vi "Array Variant to Key List.vi"(5 "section":string, 7 "Prefix":string, 8 "Error In":errorcluster, 10 "Label.Text":string, 11 "Variant":variant) -> (0 "Error Out":errorcluster, 2 "Key list":T1)   [LabVIEW 2015]
uses:
  <vilib>/Utility/Data Type/NI_Data Type.lvlib
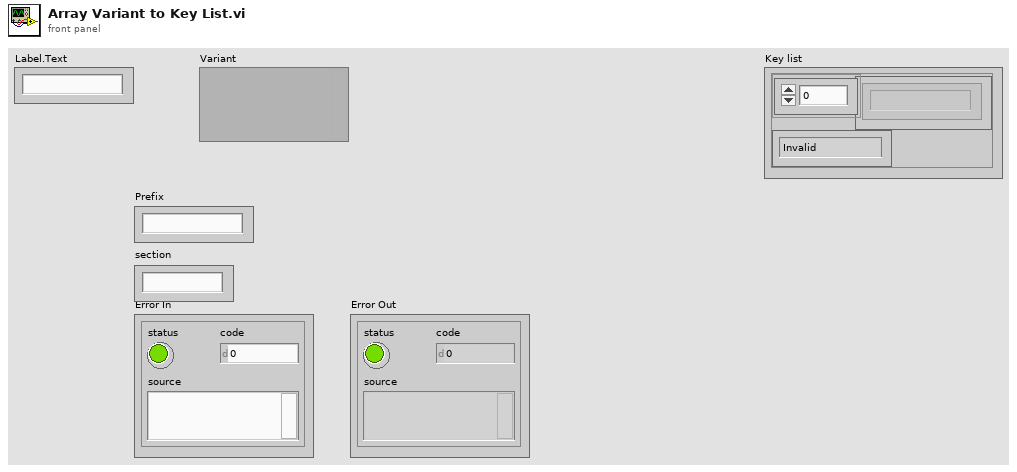
[diagram p1: front panel]
types:
  T1 = cluster{"Array":string[], "Enum":enum16{"Invalid", "Boolean", "Double", "I32", "Path", "String", "U32", "Array", "Cluster"}}
  T2 = typedef "NI_Data Type.lvlib/Data Type.ctl" = enum8{"Invalid Type", "Void", "I8", "I16", "I32", "I64", "U8", "U16", "U32", "U64", "Single Float", "Double Float", "Extended Float", "Single Complex", "Double Complex", "Extended Complex", "Enum U8", "Enum U16", "Enum U32", "Enum U64", "Single Float With Unit", "Double Float With Unit", "Extended Float With Unit", "Single Complex with Unit", "Double Complex with Unit", "Extended Complex with Unit", "Boolean", "String", "Path", "Picture", "Tag", "Array", "Cluster", "Variant", "LV Variant", "Waveform", "Timestamp", "Digital Waveform", "Digital Data", "ExpressData", "Refnum", "External Data", "VI", "Poly VI", "LabVIEW Class Instance", "Fixed Point"}
  T3 = enum16{"Invalid", "Boolean", "Double", "I32", "Path", "String", "U32", "Array", "Cluster"}
  T4 = cluster{string[], enum16{"Invalid", "Boolean", "Double", "I32", "Path", "String", "U32", "Array", "Cluster"}}
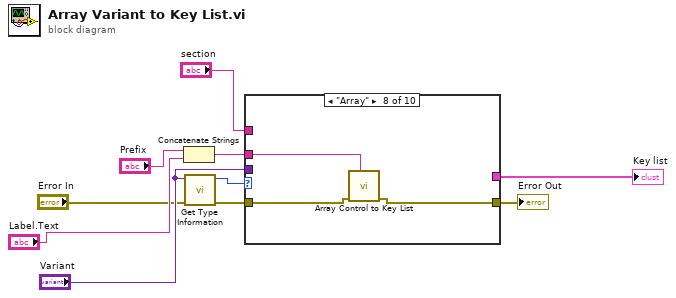
[diagram p0: block diagram]
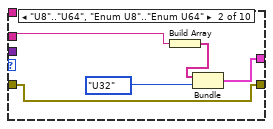
[diagram p3: hidden frame]
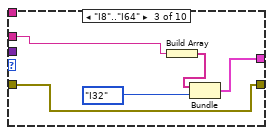
[diagram p4: hidden frame]
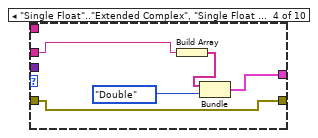
[diagram p5: hidden frame]
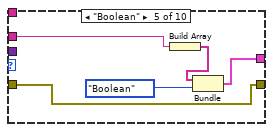
[diagram p6: hidden frame]
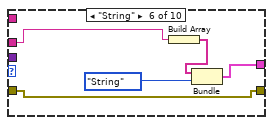
[diagram p7: hidden frame]
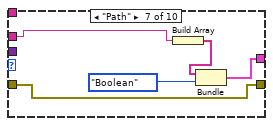
[diagram p8: hidden frame]
diagram:
  n1 = Concatenate Strings("Prefix", "Label.Text") -> (w7:string)
  n2 = call <vilib>:"Get Type Information.vi"("error in (no error)"="Error In", "Variant"="Variant") -> ("error out"=w6:errorcluster, "Type"=w10:T2)  [unwired: 5 in, 3 out]
  n3 = case shown="\"Array\"" w10 {
    tunnel: "section" -> [_ _ _ _ _ _ _ _ _ _]
    tunnel: w7 -> [_ w14 w17 w22 w31 w33 w37 w43 _ _]
    tunnel: w6 -> [w11 w12 w19 w24 w28 w34 w39 w44 _ _]
    tunnel: [w11 w12 w19 w24 w28 w34 w39 w42 _ _] -> w5
    tunnel: "Variant" -> [_ _ _ _ _ _ _ _ _ _]
    tunnel: [_ w13 w18 w23 w27 w32 w38 _ _ _] -> w4
    frame "Invalid Type", Default {
    }
    frame "U8".."U64", "Enum U8".."Enum U64" {
      n4 = Build Array(w14) -> (w16:string[])
      n5 = Bundle(w16, T3."U32") -> (w13:T4)  [unwired: 1 in]
    }
    frame "I8".."I64" {
      n6 = Build Array(w17) -> (w21:string[])
      n7 = Bundle(w21, T3."I32") -> (w18:T4)  [unwired: 1 in]
    }
    frame "Single Float".."Extended Complex", "Single Float With Unit".."Extended Complex with Unit" {
      n8 = Build Array(w22) -> (w26:string[])
      n9 = Bundle(w26, T3."Double") -> (w23:T4)  [unwired: 1 in]
    }
    frame "Boolean" {
      n10 = Build Array(w31) -> (w30:string[])
      n11 = Bundle(w30, T3."Boolean") -> (w27:T4)  [unwired: 1 in]
    }
    frame "String" {
      n12 = Build Array(w33) -> (w36:string[])
      n13 = Bundle(w36, T3."String") -> (w32:T4)  [unwired: 1 in]
    }
    frame "Path" {
      n14 = Build Array(w37) -> (w41:string[])
      n15 = Bundle(w41, T3."Boolean") -> (w38:T4)  [unwired: 1 in]
    }
    frame "Array" {
      n16 = call "Array Control to Key List.vi"("Prefix"=w43, "Error In"=w44) -> ("Error Out"=w42:errorcluster)  [unwired: 8 in, 1 out]
    }
    frame "Cluster" {
    }
    frame "Fixed Point" {
    }
  }
  "Error Out" <- w5
  "Key list" <- w4
